vi "Main.vi"() -> ()   [LabVIEW 2018] (continued)
                n2123 = Delete From Array(array=w3655, length=w3654, index=62 ("索引")) -> (deleted portion=w3669:u32[])  [unwired: 1 out]
                n2124 = To Unsigned Word Integer(number=w3675) -> (unsigned 16bit integer=w3686:u16[])
                n2125 = To Unsigned Word Integer(number=w3676) -> (unsigned 16bit integer=w3677:u16[])
                n2126 = To Unsigned Word Integer(number=w3674) -> (unsigned 16bit integer=w3691:u16[])
                n2127 = To Unsigned Word Integer(number=w3656) -> (unsigned 16bit integer=w3661:u16[])
                n2128 = To Unsigned Word Integer(number=w3669) -> (unsigned 16bit integer=w3664:u16[])
                n2129 = call "还原为字符串.vi"("输入数组"=w3677) -> ("字符串"=w3679:string)  [unwired: 9 in, 1 out]
                n2130 = call "还原为字符串.vi"("输入数组"=w3686) -> ("字符串"=w3684:string)  [unwired: 9 in, 1 out]
                n2131 = call "还原为字符串.vi"("输入数组"=w3691) -> ("字符串"=w3689:string)  [unwired: 9 in, 1 out]
                n2132 = call "还原为字符串.vi"("输入数组"=w3661) -> ("字符串"=w3659:string)  [unwired: 9 in, 1 out]
                n2133 = call "还原为字符串.vi"("输入数组"=w3664) -> ("字符串"=w3666:string)  [unwired: 9 in, 1 out]
                n2134 = Match Pattern(string=w3679, regular expression="\r" ("正则表达式")) -> (before substring=w3678:string)  [unwired: 1 in, 3 out]
                n2135 = Match Pattern(string=w3684, regular expression="\r" ("正则表达式")) -> (before substring=w3685:string)  [unwired: 1 in, 3 out]
                n2136 = Match Pattern(string=w3689, regular expression="\r" ("正则表达式")) -> (before substring=w3690:string)  [unwired: 1 in, 3 out]
                n2137 = Match Pattern(string=w3659, regular expression="\r" ("正则表达式")) -> (before substring=w3660:string)  [unwired: 1 in, 3 out]
                n2138 = Match Pattern(string=w3666, regular expression="\r" ("正则表达式")) -> (before substring=w3665:string)  [unwired: 1 in, 3 out]
                n2139 = Match Pattern(string=w3678, regular expression="\u0000" ("正则表达式")) -> (before substring=w3653:string)  [unwired: 1 in, 3 out]
                n2140 = Match Pattern(string=w3685, regular expression="\u0000" ("正则表达式")) -> (before substring=w3652:string)  [unwired: 1 in, 3 out]
                n2141 = Match Pattern(string=w3690, regular expression="\u0000" ("正则表达式")) -> (before substring=w3651:string)  [unwired: 1 in, 3 out]
                n2142 = Match Pattern(string=w3660, regular expression="\u0000" ("正则表达式")) -> (before substring=w3649:string)  [unwired: 1 in, 3 out]
                n2143 = Match Pattern(string=w3665, regular expression="\u0000" ("正则表达式")) -> (before substring=w3650:string)  [unwired: 1 in, 3 out]
                n2144 = Insert Into Array(array=string[] [] ("数组"), index=0 ("索引"), new element #1="202" ("新元素/子数组"), new element #2=w3741, new element #3=w3739, new element #4=w3740, new element #5=w3741, new element #6=w3742, new element #7=w3743, new element #8=w3744, new element #9=w3745, new element #10=w3746, new element #11=w3747, new element #12=w3653, new element #13=w3652, new element #14=w3651, new element #15=w3650, new element #16=w3649) -> (w3647:string[])
                n2145 = stacked-sequence {
                  tunnel: w3670 -> [_ w3749]
                  tunnel: [_ w3750] -> w3648
                  tunnel: w3647 -> [w3748 _]
                  frame #0 {
                    "202data" <- w3748
                  }
                  frame #1 {
                    n2146 = property on="ST202数据读取(事件)" class="Bool (严格)"("Val(Sgnl)"=TRUE ("值(信号)")) -> ()  [unwired: 2 in, 2 out]
                    n2147 = disable-structure shown="禁用" {
                      disable-tunnel: w3749 -> [w3753 w3755]
                      disable-tunnel: [w3752 w3755] -> w3750
                      frame Disabled {
                        n2148 = property on="ST202画曲线" class="Bool (严格)"(error in=w3753, "Val(Sgnl)"=TRUE ("值(信号)")) -> (error out=w3752:errorcluster)  [unwired: 1 in, 1 out]
                      }
                      frame Enabled {
                      }
                    }
                  }
                }
              }
            }
          }
          frame "写" {
            w3914 = u8 132 items=["I/O (P)"=128, "Input (I)"=129, "Output (Q)"=130, "Bit Memory (M)"=131, "Data (DB)"=132, "Instance Data (DI)"=133, "Local Data (L)"=134, "Predecessor Local Data (VL)"=135] ("寄存器类型")
            w3913 = u16 1 items=["byte", "word", "Dword"] ("数据类型")
            w3931 = u8 132 items=["I/O (P)"=128, "Input (I)"=129, "Output (Q)"=130, "Bit Memory (M)"=131, "Data (DB)"=132, "Instance Data (DI)"=133, "Local Data (L)"=134, "Predecessor Local Data (VL)"=135] ("寄存器类型")
            w3932 = u16 1 items=["byte", "word", "Dword"] ("数据类型")
            w3939 = u8 132 items=["I/O (P)"=128, "Input (I)"=129, "Output (Q)"=130, "Bit Memory (M)"=131, "Data (DB)"=132, "Instance Data (DI)"=133, "Local Data (L)"=134, "Predecessor Local Data (VL)"=135] ("寄存器类型")
            w3940 = u16 1 items=["byte", "word", "Dword"] ("数据类型")
            w3942 = u8 132 items=["I/O (P)"=128, "Input (I)"=129, "Output (Q)"=130, "Bit Memory (M)"=131, "Data (DB)"=132, "Instance Data (DI)"=133, "Local Data (L)"=134, "Predecessor Local Data (VL)"=135] ("寄存器类型")
            w3941 = u16 1 items=["byte", "word", "Dword"] ("数据类型")
            w3948 = u8 132 items=["I/O (P)"=128, "Input (I)"=129, "Output (Q)"=130, "Bit Memory (M)"=131, "Data (DB)"=132, "Instance Data (DI)"=133, "Local Data (L)"=134, "Predecessor Local Data (VL)"=135] ("寄存器类型")
            w3945 = u16 1 items=["byte", "word", "Dword"] ("数据类型")
            n2149 = local read "20看门狗"() -> (w3924:i32)
            n2150 = case shown="0" w3924 {
              tunnel: [0 ("y") 1 ("y")] -> w3923
              frame 1, Default {
              }
              frame 0 {
              }
            }
            "20看门狗" <- w3923
            n2151 = call "S7_Write.vi"("TCP"=w3906, "寄存器类型"=w3948, "DB #"=u16 20, "写入地址"=u32 2, "数据类型"=w3945, "写入数据"=w3923) -> ("TCP"=w3922:refnum<k5>, "error out"=w3921:errorcluster)  [unwired: 7 in, 1 out]
            n2152 = case shown="假" "201扫码回复写入" {
              tunnel: w3922 -> [w3976 w3984]
              tunnel: w3921 -> [w3975 w3983]
              tunnel: [w3976 w3980] -> w3919
              tunnel: [w3975 w3979] -> w3918
              tunnel: [999 w3977] -> w3917
              frame False {
              }
              frame True {
                w3992 = u8 132 items=["I/O (P)"=128, "Input (I)"=129, "Output (Q)"=130, "Bit Memory (M)"=131, "Data (DB)"=132, "Instance Data (DI)"=133, "Local Data (L)"=134, "Predecessor Local Data (VL)"=135] ("寄存器类型")
                w3991 = u16 1 items=["byte", "word", "Dword"] ("数据类型")
                w3986 = u8 132 items=["I/O (P)"=128, "Input (I)"=129, "Output (Q)"=130, "Bit Memory (M)"=131, "Data (DB)"=132, "Instance Data (DI)"=133, "Local Data (L)"=134, "Predecessor Local Data (VL)"=135] ("寄存器类型")
                w3987 = u16 1 items=["byte", "word", "Dword"] ("数据类型")
                n2153 = local read "上一站号 (201)"() -> (w3982:string)
                n2154 = local read "上一站结果 (201)"() -> (w3981:string)
                n2155 = Decimal String To Number(string=w3982, default (0L)=u32 0 ("默认(0 I32)")) -> (number=w3996:u32)  [unwired: 1 in, 1 out]
                n2156 = call "S7_Write.vi"("TCP"=w3984, "寄存器类型"=w3986, "DB #"=u16 20, "写入地址"=u32 12, "数据类型"=w3987, "写入数据"=w3996, "error in"=w3983) -> ("TCP"=w3995:refnum<k5>, "error out"=w3994:errorcluster)  [unwired: 6 in, 1 out]
                n2157 = Equal?(x=w3981, y="OK") -> (x = y?=w3998:bool)
                n2158 = case shown="假" w3998 {
                  tunnel: [u32 2 ("写入数据") u32 1 ("写入数据")] -> w3999
                  frame False {
                  }
                  frame True {
                  }
                }
                n2159 = local read "扫码请求回复201"() -> (w3978:string)
                n2160 = call "S7_Write.vi"("TCP"=w3995, "寄存器类型"=w3992, "DB #"=u16 20, "写入地址"=u32 14, "数据类型"=w3991, "写入数据"=w3999, "error in"=w3994) -> ("TCP"=w3980:refnum<k5>, "error out"=w3979:errorcluster)  [unwired: 6 in, 1 out]
                n2161 = Decimal String To Number(string=w3978) -> (number=w3977:i32)  [unwired: 2 in, 1 out]
              }
            }
            n2162 = call "S7_Write.vi"("TCP"=w3919, "寄存器类型"=w3942, "DB #"=u16 20, "写入地址"=u32 4, "数据类型"=w3941, "写入数据"=w3917, "error in"=w3918) -> ("TCP"=w3912:refnum<k5>, "error out"=w3911:errorcluster)  [unwired: 6 in, 1 out]
            n2163 = case shown="真" "201数据回复写入" {
              tunnel: [999 w3972] -> w3910
              frame False {
              }
              frame True {
                n2164 = local read "数据保存请求回复201"() -> (w3973:string)
                n2165 = Decimal String To Number(string=w3973) -> (number=w3972:i32)  [unwired: 2 in, 1 out]
              }
            }
            n2166 = call "S7_Write.vi"("TCP"=w3912, "寄存器类型"=w3914, "DB #"=u16 20, "写入地址"=u32 6, "数据类型"=w3913, "写入数据"=w3910, "error in"=w3911) -> ("TCP"=w3908:refnum<k5>, "error out"=w3907:errorcluster)  [unwired: 6 in, 1 out]
            n2167 = case shown="真" "202扫码回复写入" {
              tunnel: [999 w4008] -> w3935
              tunnel: w3908 -> [w4006 w4025]
              tunnel: w3907 -> [w4005 w4024]
              tunnel: [w4006 w4013] -> w3934
              tunnel: [w4005 w4012] -> w3933
              frame False {
              }
              frame True {
                w4019 = u8 132 items=["I/O (P)"=128, "Input (I)"=129, "Output (Q)"=130, "Bit Memory (M)"=131, "Data (DB)"=132, "Instance Data (DI)"=133, "Local Data (L)"=134, "Predecessor Local Data (VL)"=135] ("寄存器类型")
                w4020 = u16 1 items=["byte", "word", "Dword"] ("数据类型")
                w4027 = u8 132 items=["I/O (P)"=128, "Input (I)"=129, "Output (Q)"=130, "Bit Memory (M)"=131, "Data (DB)"=132, "Instance Data (DI)"=133, "Local Data (L)"=134, "Predecessor Local Data (VL)"=135] ("寄存器类型")
                w4026 = u16 1 items=["byte", "word", "Dword"] ("数据类型")
                n2168 = local read "上一站号 (202)"() -> (w4011:string)
                n2169 = Decimal String To Number(string=w4011) -> (number=w4023:i32)  [unwired: 2 in, 1 out]
                n2170 = call "S7_Write.vi"("TCP"=w4025, "寄存器类型"=w4027, "DB #"=u16 20, "写入地址"=u32 16, "数据类型"=w4026, "写入数据"=w4023, "error in"=w4024) -> ("TCP"=w4015:refnum<k5>, "error out"=w4016:errorcluster)  [unwired: 6 in, 1 out]
                n2171 = local read "上一站结果 (202)"() -> (w4010:string)
                n2172 = local read "扫码请求回复202"() -> (w4009:string)
                n2173 = Equal?(x=w4010, y="OK") -> (x = y?=w4022:bool)
                n2174 = case shown="假" w4022 {
                  tunnel: [u32 2 ("写入数据") u32 1 ("写入数据")] -> w4014
                  frame False {
                  }
                  frame True {
                  }
                }
                n2175 = call "S7_Write.vi"("TCP"=w4015, "寄存器类型"=w4019, "DB #"=u16 20, "写入地址"=u32 18, "数据类型"=w4020, "写入数据"=w4014, "error in"=w4016) -> ("TCP"=w4013:refnum<k5>, "error out"=w4012:errorcluster)  [unwired: 6 in, 1 out]
                n2176 = Decimal String To Number(string=w4009) -> (number=w4008:i32)  [unwired: 2 in, 1 out]
              }
            }
            n2177 = call "S7_Write.vi"("TCP"=w3934, "寄存器类型"=w3939, "DB #"=u16 20, "写入地址"=u32 8, "数据类型"=w3940, "写入数据"=w3935, "error in"=w3933) -> ("TCP"=w3927:refnum<k5>, "error out"=w3928:errorcluster)  [unwired: 6 in, 1 out]
            n2178 = case shown="假" "202数据回复写入" {
              tunnel: [999 w4004] -> w3925
              frame False {
              }
              frame True {
                n2179 = local read "数据保存请求回复202"() -> (w4003:string)
                n2180 = Decimal String To Number(string=w4003) -> (number=w4004:i32)  [unwired: 2 in, 1 out]
              }
            }
            n2181 = call "S7_Write.vi"("TCP"=w3927, "寄存器类型"=w3931, "DB #"=u16 20, "写入地址"=u32 10, "数据类型"=w3932, "写入数据"=w3925, "error in"=w3928) -> ("TCP"=w3905:refnum<k5>, "error out"=w3903:errorcluster)  [unwired: 6 in, 1 out]
            n2182 = disable-structure shown="启用" {
              disable-tunnel: w3905 -> [w3951 w3967]
              disable-tunnel: [w3951 w3959] -> w3904
              disable-tunnel: w3903 -> [w3952 w3958]
              disable-tunnel: [w3952 w3956] -> w3902
              disable-tunnel: [_ w3954] -> w3901
              disable-tunnel: [_ w3953] -> w3900
              frame Disabled {
              }
              frame Enabled {
                w3965 = u16 20 ("DB #")
                w3964 = u8 132 items=["I/O (P)"=128, "Input (I)"=129, "Output (Q)"=130, "Bit Memory (M)"=131, "Data (DB)"=132, "Instance Data (DI)"=133, "Local Data (L)"=134, "Predecessor Local Data (VL)"=135] ("寄存器类型")
                w3963 = u16 1 items=["byte", "word", "Dword"] ("数据类型")
                n2183 = call "S7_Read.vi"("TCP"=w3967, "DB #"=w3965, "读取长度"=u16 1, "寄存器类型"=w3964, "起始地址"=u32 264 ("写入地址"), "数据类型"=w3963, "error in"=w3958) -> ("TCP"=w3966:refnum<k5>, "数据"=w3960:u32[], "error out"=w3957:errorcluster)  [unwired: 5 in, 1 out]
                n2184 = Index Array(array=w3960) -> (element=w3953:u32)  [unwired: 1 in]
                n2185 = case shown="1" w3953 {
                  tunnel: ["未选择" "LF37G" "LF37.1G"] -> w3954
                  frame 0, Default {
                  }
                  frame 1 {
                  }
                  frame 2 {
                  }
                }
                n2186 = call "S7_Write.vi"("TCP"=w3966, "寄存器类型"=w3964, "DB #"=w3965, "写入地址"=u32 266, "数据类型"=w3963, "写入数据"=w3953, "error in"=w3957) -> ("TCP"=w3959:refnum<k5>, "error out"=w3956:errorcluster)  [unwired: 6 in, 1 out]
              }
            }
            n2187 = local write "产品型号"(w3900) -> ()
            n2188 = local write "产品型号20-90"(w3901) -> ()
          }
          frame "错误" {
            n2189 = call "S7_Close.vi"("TCP Connection Ref"=w4036) -> ("error out"=w4037:errorcluster)  [unwired: 10 in]
            n2190 = call <vilib>:"Clear Errors.vi"("error in (no error)"=w4037) -> ()  [unwired: 5 in, 2 out]
          }
          frame "退出" {
            n2191 = call "S7_Close.vi"("TCP Connection Ref"=w4043) -> ("error out"=w4044:errorcluster)  [unwired: 10 in]
            n2192 = call <vilib>:"Clear Errors.vi"("error in (no error)"=w4044) -> ()  [unwired: 5 in, 2 out]
          }
        }
      }
      n2193 = while {
        shift-right: [w1194] -> _
        shift-left: errorcluster {"status"=FALSE, "code"=0, "source"=""} ("错误常量") -> [w1197]
        shift-right: [w1193] -> _
        shift-left: enum16{"初始化", "读", "写", "错误", "退出"}."初始化" -> [w1198]
        shift-right: [w1195] -> _
        shift-left: _ -> [w1192]
        stop <- w1191 stop-if-true
        n2194 = local read "退出"() -> (w1199:bool)
        n2195 = case shown="假" w1199 {
          tunnel: w1198 -> [w1200 _]
          tunnel: [w1201 enum16{"初始化", "读", "写", "错误", "退出"}."退出"] -> w1190
          tunnel: w1197 -> [w1202 _]
          frame False {
            n2196 = case shown="错误" w1202 {
              tunnel: [w1203 enum16{"初始化", "读", "写", "错误", "退出"}."错误"] -> w1201
              tunnel: w1200 -> [w1203 _]
              frame No Error {
              }
              frame Error {
              }
            }
          }
          frame True {
          }
        }
        n2197 = Wait (ms)(milliseconds to wait=u32 80 ("等待时间（毫秒）")) -> ()  [unwired: 1 out]
        n2198 = case shown="\"写\"" w1190 {
          tunnel: [w1206 w1258 w1567 refnum<k5> refnum ("TCP") refnum<k5> refnum ("TCP")] -> w1195
          tunnel: [w1207 w1257 w1565 errorcluster {"status"=FALSE, "code"=0, "source"=""} ("error out") errorcluster {"status"=FALSE, "code"=0, "source"=""} ("error out")] -> w1194
          tunnel: [enum16{"初始化", "读", "写", "错误", "退出"}."读" enum16{"初始化", "读", "写", "错误", "退出"}."写" enum16{"初始化", "读", "写", "错误", "退出"}."读" enum16{"初始化", "读", "写", "错误", "退出"}."初始化" enum16{"初始化", "读", "写", "错误", "退出"}."退出"] -> w1193
          tunnel: w1192 -> [_ w1289 w1625 w1738 w1745]
          tunnel: [FALSE FALSE FALSE FALSE TRUE] -> w1191
          frame "初始化", Default {
            w1219 = u16 0 items=["byte", "word", "Dword"] ("数据类型")
            w1217 = u8 132 items=["I/O (P)"=128, "Input (I)"=129, "Output (Q)"=130, "Bit Memory (M)"=131, "Data (DB)"=132, "Instance Data (DI)"=133, "Local Data (L)"=134, "Predecessor Local Data (VL)"=135] ("寄存器类型")
            w1230 = u16 0 items=["byte", "word", "Dword"] ("数据类型")
            w1232 = u8 132 items=["I/O (P)"=128, "Input (I)"=129, "Output (Q)"=130, "Bit Memory (M)"=131, "Data (DB)"=132, "Instance Data (DI)"=133, "Local Data (L)"=134, "Predecessor Local Data (VL)"=135] ("寄存器类型")
            w1221 = u16 0 items=["byte", "word", "Dword"] ("数据类型")
            w1223 = u8 132 items=["I/O (P)"=128, "Input (I)"=129, "Output (Q)"=130, "Bit Memory (M)"=131, "Data (DB)"=132, "Instance Data (DI)"=133, "Local Data (L)"=134, "Predecessor Local Data (VL)"=135] ("寄存器类型")
            w1245 = u8 0 items=["S7-1200.200.200SMART"=0, "S7-300"=2, "S7-400"=3] ("PLC 系列")
            n2199 = call "S7_Open.vi"("IP 地址"="192.168.1.60", "PLC 系列"=w1245, "超时（MS）"=100) -> ("TCP"=w1209:refnum<k5>, "error out"=w1208:errorcluster)  [unwired: 10 in, 1 out]
            n2200 = case shown="错误" w1208 {
              tunnel: [FALSE TRUE] -> w1241
              frame No Error {
              }
              frame Error {
              }
            }
            n2201 = local write "ST60通讯状态"(w1241) -> ()
            n2202 = call "S7_Read.vi"("TCP"=w1209, "DB #"=u16 20, "读取长度"=u16 13, "寄存器类型"=w1223, "起始地址"=u32 52, "数据类型"=w1221, "error in"=w1208) -> ("TCP"=w1238:refnum<k5>, "数据"=w1226:u32[], "error out"=w1228:errorcluster)  [unwired: 5 in, 1 out]
            n2203 = To Unsigned Word Integer(number=w1226) -> (unsigned 16bit integer=w1227:u16[])
            n2204 = call "还原为字符串.vi"("error in (no error)"=w1228, "输入数组"=w1227) -> ("error out"=w1239:errorcluster, "字符串"=w1229:string)  [unwired: 8 in]
            n2205 = local write "602二维码"(w1229) -> ()
            n2206 = call "S7_Read.vi"("TCP"=w1238, "DB #"=u16 20, "读取长度"=u16 13, "寄存器类型"=w1232, "起始地址"=u32 74, "数据类型"=w1230, "error in"=w1239) -> ("TCP"=w1211:refnum<k5>, "数据"=w1235:u32[], "error out"=w1237:errorcluster)  [unwired: 5 in, 1 out]
            n2207 = To Unsigned Word Integer(number=w1235) -> (unsigned 16bit integer=w1236:u16[])
            n2208 = call "还原为字符串.vi"("error in (no error)"=w1237, "输入数组"=w1236) -> ("error out"=w1210:errorcluster, "字符串"=w1240:string)  [unwired: 8 in]
            n2209 = local write "603二维码"(w1240) -> ()
            n2210 = call "S7_Read.vi"("TCP"=w1211, "DB #"=u16 20, "读取长度"=u16 13, "寄存器类型"=w1217, "起始地址"=u32 30, "数据类型"=w1219, "error in"=w1210) -> ("TCP"=w1206:refnum<k5>, "数据"=w1214:u32[], "error out"=w1212:errorcluster)  [unwired: 5 in, 1 out]
            n2211 = To Unsigned Word Integer(number=w1214) -> (unsigned 16bit integer=w1213:u16[])
            n2212 = call "还原为字符串.vi"("error in (no error)"=w1212, "输入数组"=w1213) -> ("error out"=w1207:errorcluster, "字符串"=w1220:string)  [unwired: 8 in]
            n2213 = local write "601二维码"(w1220) -> ()
          }
          frame "读" {
            w1290 = u16 0 items=["byte", "word", "Dword"] ("数据类型")
            w1292 = u8 132 items=["I/O (P)"=128, "Input (I)"=129, "Output (Q)"=130, "Bit Memory (M)"=131, "Data (DB)"=132, "Instance Data (DI)"=133, "Local Data (L)"=134, "Predecessor Local Data (VL)"=135] ("寄存器类型")
            n2214 = call "S7_Read.vi"("TCP"=w1289, "DB #"=u16 20, "读取长度"=u16 1, "寄存器类型"=w1292, "起始地址"=u32 0, "数据类型"=w1290) -> ("TCP"=w1287:refnum<k5>, "数据"=w1297:u32[], "读取成功"=w1300:bool, "error out"=w1286:errorcluster)  [unwired: 6 in]
            n2215 = Not(x=w1300) -> (.not. x?=→"ST60通讯状态":bool)
            n2216 = Index Array(array=w1297, index=0 ("索引")) -> (element=w1298:u32)
            n2217 = Number To Boolean Array(number=w1298) -> (Boolean array=w1299:bool[])
            n2218 = Index Array(array=w1299, index #1=0 ("索引")) -> (element #1=w1267:bool, element #2=w1256:bool, element #3=w1255:bool, element #4=w1252:bool, element #5=w1251:bool, element #6=w1249:bool)  [unwired: 5 in]
            "ST601扫码请求" <- w1267
            "ST601数据读取" <- w1256
            "ST602扫码请求" <- w1255
            "ST602数据读取" <- w1252
            "ST603扫码请求" <- w1251
            "ST603数据读取" <- w1249
            n2219 = disable-structure shown="启用" {
              disable-tunnel: [w1312 w1314] -> w1269
              disable-tunnel: w1267 -> [w1311 w1314]
              frame Disabled {
                n2220 = call <vilib>:"Boolean Crossing PtByPt.vi"("direction"=enum16{"either", "false-true", "true-false"}."true-false", "input"=w1311) -> ("crossing"=w1312:bool)  [unwired: 1 in]
              }
              frame Enabled {
              }
            }
            n2221 = call <vilib>:"Boolean Crossing PtByPt.vi"("direction"=enum16{"either", "false-true", "true-false"}."false-true", "input"=w1267) -> ("crossing"=w1285:bool)  [unwired: 1 in]
            n2222 = case shown="真" w1285 {
              tunnel: w1287 -> [w1546 w1551]
              tunnel: w1286 -> [w1545 w1552]
              tunnel: [w1546 w1550] -> w1284
              tunnel: [w1545 w1548] -> w1283
              frame False {
              }
              frame True {
                w1560 = u16 0 items=["byte", "word", "Dword"] ("数据类型")
                w1558 = u8 132 items=["I/O (P)"=128, "Input (I)"=129, "Output (Q)"=130, "Bit Memory (M)"=131, "Data (DB)"=132, "Instance Data (DI)"=133, "Local Data (L)"=134, "Predecessor Local Data (VL)"=135] ("寄存器类型")
                n2223 = call "S7_Read.vi"("TCP"=w1551, "DB #"=u16 20, "读取长度"=u16 13, "寄存器类型"=w1558, "起始地址"=u32 30, "数据类型"=w1560, "error in"=w1552) -> ("TCP"=w1550:refnum<k5>, "数据"=w1555:u32[], "error out"=w1553:errorcluster)  [unwired: 5 in, 1 out]
                n2224 = To Unsigned Word Integer(number=w1555) -> (unsigned 16bit integer=w1554:u16[])
                n2225 = call "还原为字符串.vi"("error in (no error)"=w1553, "输入数组"=w1554) -> ("error out"=w1549:errorcluster, "字符串"=w1547:string)  [unwired: 8 in]
                n2226 = stacked-sequence {
                  tunnel: w1549 -> [_ w1563]
                  tunnel: [_ w1562] -> w1548
                  tunnel: w1547 -> [w1561 _]
                  frame #0 {
                    "601二维码" <- w1561
                  }
                  frame #1 {
                    n2227 = property on="ST601扫码请求（事件）" class="Bool (严格)"(error in=w1563, "Val(Sgnl)"=TRUE ("值(信号)")) -> (error out=w1562:errorcluster)  [unwired: 1 in, 1 out]
                  }
                }
              }
            }
            n2228 = case shown="假" w1269 {
              frame False {
                n2229 = local write "601扫码回复输入"(FALSE ("301扫码回复输入")) -> ()
              }
              frame True {
              }
            }
            n2230 = call <vilib>:"Boolean Crossing PtByPt.vi"("direction"=enum16{"either", "false-true", "true-false"}."false-true", "input"=w1256) -> ("crossing"=w1281:bool)  [unwired: 1 in]
            n2231 = disable-structure shown="启用" {
              disable-tunnel: enum16{"either", "false-true", "true-false"}."true-false" ("direction") -> [w1325 _]
              disable-tunnel: [w1324 w1326] -> w1278
              disable-tunnel: w1256 -> [w1323 w1326]
              frame Disabled {
                n2232 = call <vilib>:"Boolean Crossing PtByPt.vi"("direction"=w1325, "input"=w1323) -> ("crossing"=w1324:bool)  [unwired: 1 in]
              }
              frame Enabled {
              }
            }
            n2233 = case shown="真" w1281 {
              tunnel: [w1505 w1515] -> w1276
              tunnel: [w1504 w1507] -> w1275
              tunnel: w1283 -> [w1504 w1511]
              tunnel: w1284 -> [w1505 w1512]
              frame False {
              }
              frame True {
                w1524 = u16 1 items=["byte", "word", "Dword"] ("数据类型")
                w1526 = u8 132 items=["I/O (P)"=128, "Input (I)"=129, "Output (Q)"=130, "Bit Memory (M)"=131, "Data (DB)"=132, "Instance Data (DI)"=133, "Local Data (L)"=134, "Predecessor Local Data (VL)"=135] ("寄存器类型")
                w1519 = u16 1 items=["byte", "word", "Dword"] ("数据类型")
                w1521 = u8 132 items=["I/O (P)"=128, "Input (I)"=129, "Output (Q)"=130, "Bit Memory (M)"=131, "Data (DB)"=132, "Instance Data (DI)"=133, "Local Data (L)"=134, "Predecessor Local Data (VL)"=135] ("寄存器类型")
                n2234 = call "S7_Read.vi"("TCP"=w1512, "DB #"=u16 20, "读取长度"=u16 1, "寄存器类型"=w1521, "起始地址"=u32 94, "数据类型"=w1519, "error in"=w1511) -> ("TCP"=w1532:refnum<k5>, "数据"=w1534:u32[], "error out"=w1533:errorcluster)  [unwired: 5 in, 1 out]
                n2235 = Index Array(array=w1534) -> (element=w1536:u32)  [unwired: 1 in]
                n2236 = Equal?(x=w1536, y=u32 1) -> (x = y?=w1535:bool)
                n2237 = case shown="真" w1535 {
                  tunnel: ["NG" "OK"] -> w1510
                  frame False {
                  }
                  frame True {
                  }
                }
                n2238 = call "S7_Read.vi"("TCP"=w1532, "DB #"=u16 20, "读取长度"=u16 1, "寄存器类型"=w1526, "起始地址"=u32 100, "数据类型"=w1524, "error in"=w1533) -> ("TCP"=w1515:refnum<k5>, "数据"=w1514:u32[], "error out"=w1508:errorcluster)  [unwired: 5 in, 1 out]
                n2239 = Index Array(array=w1514) -> (element=w1513:u32)  [unwired: 1 in]
                n2240 = Number To Decimal String(number=w1513) -> (decimal integer string=w1509:string)  [unwired: 1 in]
                n2241 = Format Date/Time String(time format string (%c)="%Y-%m-%d" ("时间格式字符串(%c)")) -> (date/time string=w1537:string)  [unwired: 2 in]
                n2242 = Get Date/Time String(want seconds? (F)=TRUE ("需要秒？(F)")) -> (time string=w1538:string)  [unwired: 2 in, 1 out]
                n2243 = Insert Into Array(array=string[] [] ("数组"), index=0 ("索引"), new element #1="601" ("新元素/子数组"), new element #2=w1510, new element #3=w1537, new element #4=w1538, new element #5=w1510, new element #6=w1509) -> (w1506:string[])
                n2244 = stacked-sequence {
                  tunnel: w1508 -> [_ w1542]
                  tunnel: [_ w1541] -> w1507
                  tunnel: w1506 -> [w1539 _]
                  frame #0 {
                    "601数据" <- w1539
                  }
                  frame #1 {
                    n2245 = property on="ST601数据读取（事件）" class="Bool (严格)"(error in=w1542, "Val(Sgnl)"=TRUE ("值(信号)")) -> (error out=w1541:errorcluster)  [unwired: 1 in, 1 out]
                  }
                }
              }
            }
            n2246 = case shown="假" w1278 {
              frame False {
                n2247 = local write "601数据回复输入"(FALSE ("301数据回复输入")) -> ()
              }
              frame True {
              }
            }
            n2248 = disable-structure shown="启用" {
              disable-tunnel: [w1309 w1310] -> w1277
              disable-tunnel: w1255 -> [w1307 w1310]
              frame Disabled {
                n2249 = call <vilib>:"Boolean Crossing PtByPt.vi"("direction"=enum16{"either", "false-true", "true-false"}."true-false", "input"=w1307) -> ("crossing"=w1309:bool)  [unwired: 1 in]
              }
              frame Enabled {
              }
            }
            n2250 = case shown="假" w1277 {
              frame False {
                n2251 = local write "602扫码回复输入"(FALSE ("302扫码回复输入")) -> ()
              }
              frame True {
              }
            }
            n2252 = disable-structure shown="启用" {
              disable-tunnel: [w1320 w1322] -> w1254
              disable-tunnel: w1252 -> [w1319 w1322]
              frame Disabled {
                n2253 = call <vilib>:"Boolean Crossing PtByPt.vi"("direction"=enum16{"either", "false-true", "true-false"}."true-false", "input"=w1319) -> ("crossing"=w1320:bool)  [unwired: 1 in]
              }
              frame Enabled {
              }
            }
            n2254 = case shown="假" w1254 {
              frame False {
                n2255 = local write "602数据回复输入"(FALSE ("302数据回复输入")) -> ()
              }
              frame True {
              }
            }
            n2256 = disable-structure shown="启用" {
              disable-tunnel: [w1305 w1306] -> w1253
              disable-tunnel: w1251 -> [w1303 w1306]
              frame Disabled {
                n2257 = call <vilib>:"Boolean Crossing PtByPt.vi"("direction"=enum16{"either", "false-true", "true-false"}."true-false", "input"=w1303) -> ("crossing"=w1305:bool)  [unwired: 1 in]
              }
              frame Enabled {
              }
            }
            n2258 = call <vilib>:"Boolean Crossing PtByPt.vi"("direction"=enum16{"either", "false-true", "true-false"}."false-true", "input"=w1255) -> ("crossing"=w1274:bool)  [unwired: 1 in]
            n2259 = case shown="真" w1274 {
              tunnel: w1276 -> [w1482 w1488]
              tunnel: w1275 -> [w1481 w1487]
              tunnel: [w1481 w1484] -> w1272
              tunnel: [w1482 w1486] -> w1273
              frame False {
              }
              frame True {
                w1489 = u16 0 items=["byte", "word", "Dword"] ("数据类型")
                w1491 = u8 132 items=["I/O (P)"=128, "Input (I)"=129, "Output (Q)"=130, "Bit Memory (M)"=131, "Data (DB)"=132, "Instance Data (DI)"=133, "Local Data (L)"=134, "Predecessor Local Data (VL)"=135] ("寄存器类型")
                n2260 = call "S7_Read.vi"("TCP"=w1488, "DB #"=u16 20, "读取长度"=u16 13, "寄存器类型"=w1491, "起始地址"=u32 52, "数据类型"=w1489, "error in"=w1487) -> ("TCP"=w1486:refnum<k5>, "数据"=w1494:u32[], "error out"=w1496:errorcluster)  [unwired: 5 in, 1 out]
                n2261 = To Unsigned Word Integer(number=w1494) -> (unsigned 16bit integer=w1495:u16[])
                n2262 = call "还原为字符串.vi"("error in (no error)"=w1496, "输入数组"=w1495) -> ("error out"=w1485:errorcluster, "字符串"=w1483:string)  [unwired: 8 in]
                n2263 = stacked-sequence {
                  tunnel: w1485 -> [_ w1500]
                  tunnel: [_ w1499] -> w1484
                  tunnel: w1483 -> [w1497 _]
                  frame #0 {
                    "602二维码" <- w1497
                  }
                  frame #1 {
                    n2264 = property on="ST602扫码请求 （事件）" class="Bool (严格)"(error in=w1500, "Val(Sgnl)"=TRUE ("值(信号)")) -> (error out=w1499:errorcluster)  [unwired: 1 in, 1 out]
                  }
                }
              }
            }
            n2265 = case shown="假" w1253 {
              frame False {
                n2266 = local write "603扫码回复输入"(FALSE ("303扫码回复输入")) -> ()
              }
              frame True {
              }
            }
            n2267 = disable-structure shown="启用" {
              disable-tunnel: [w1316 w1318] -> w1250
              disable-tunnel: w1249 -> [w1315 w1318]
              frame Disabled {
                n2268 = call <vilib>:"Boolean Crossing PtByPt.vi"("direction"=enum16{"either", "false-true", "true-false"}."true-false", "input"=w1315) -> ("crossing"=w1316:bool)  [unwired: 1 in]
              }
              frame Enabled {
              }
            }
            n2269 = case shown="假" w1250 {
              frame False {
                n2270 = local write "603数据回复输入"(FALSE ("303数据回复输入")) -> ()
              }
              frame True {
              }
            }
            n2271 = call <vilib>:"Boolean Crossing PtByPt.vi"("direction"=enum16{"either", "false-true", "true-false"}."false-true", "input"=w1252) -> ("crossing"=w1270:bool)  [unwired: 1 in]
            n2272 = case shown="真" w1270 {
              tunnel: w1273 -> [w1441 w1447]
              tunnel: w1272 -> [w1440 w1446]
              tunnel: [w1441 w1445] -> w1264
              tunnel: [w1440 w1443] -> w1263
              frame False {
              }
              frame True {
                w1453 = u16 1 items=["byte", "word", "Dword"] ("数据类型")
                w1455 = u8 132 items=["I/O (P)"=128, "Input (I)"=129, "Output (Q)"=130, "Bit Memory (M)"=131, "Data (DB)"=132, "Instance Data (DI)"=133, "Local Data (L)"=134, "Predecessor Local Data (VL)"=135] ("寄存器类型")
                w1448 = u16 1 items=["byte", "word", "Dword"] ("数据类型")
                w1450 = u8 132 items=["I/O (P)"=128, "Input (I)"=129, "Output (Q)"=130, "Bit Memory (M)"=131, "Data (DB)"=132, "Instance Data (DI)"=133, "Local Data (L)"=134, "Predecessor Local Data (VL)"=135] ("寄存器类型")
                n2273 = call "S7_Read.vi"("TCP"=w1447, "DB #"=u16 20, "读取长度"=u16 1, "寄存器类型"=w1450, "起始地址"=u32 102, "数据类型"=w1448, "error in"=w1446) -> ("TCP"=w1464:refnum<k5>, "数据"=w1466:u32[], "error out"=w1465:errorcluster)  [unwired: 5 in, 1 out]
                n2274 = Index Array(array=w1466) -> (element=w1467:u32)  [unwired: 1 in]
                n2275 = Number To Decimal String(number=w1467) -> (decimal integer string=w1474:string)  [unwired: 1 in]
                n2276 = call "S7_Read.vi"("TCP"=w1464, "DB #"=u16 20, "读取长度"=u16 1, "寄存器类型"=w1455, "起始地址"=u32 96, "数据类型"=w1453, "error in"=w1465) -> ("TCP"=w1445:refnum<k5>, "数据"=w1468:u32[], "error out"=w1444:errorcluster)  [unwired: 5 in, 1 out]
                n2277 = Index Array(array=w1468) -> (element=w1470:u32)  [unwired: 1 in]
                n2278 = Equal?(x=w1470, y=u32 1) -> (x = y?=w1469:bool)
                n2279 = case shown="真" w1469 {
                  tunnel: ["NG" "OK"] -> w1473
                  frame False {
                  }
                  frame True {
                  }
                }
                n2280 = Format Date/Time String(time format string (%c)="%Y-%m-%d" ("时间格式字符串(%c)")) -> (date/time string=w1471:string)  [unwired: 2 in]
                n2281 = Get Date/Time String(want seconds? (F)=TRUE ("需要秒？(F)")) -> (time string=w1472:string)  [unwired: 2 in, 1 out]
                n2282 = Insert Into Array(array=string[] [] ("数组"), index=0 ("索引"), new element #1="602" ("新元素/子数组"), new element #2=w1473, new element #3=w1471, new element #4=w1472, new element #5=w1473, new element #6=w1474) -> (w1442:string[])
                n2283 = stacked-sequence {
                  tunnel: w1444 -> [_ w1478]
                  tunnel: [_ w1477] -> w1443
                  tunnel: w1442 -> [w1475 _]
                  frame #0 {
                    "602data" <- w1475
                  }
                  frame #1 {
                    n2284 = property on="ST602数据读取（事件）" class="Bool (严格)"(error in=w1478, "Val(Sgnl)"=TRUE ("值(信号)")) -> (error out=w1477:errorcluster)  [unwired: 1 in, 1 out]
                  }
                }
              }
            }
            n2285 = call <vilib>:"Boolean Crossing PtByPt.vi"("direction"=enum16{"either", "false-true", "true-false"}."false-true", "input"=w1251) -> ("crossing"=w1266:bool)  [unwired: 1 in]
            n2286 = case shown="真" w1266 {
              tunnel: w1264 -> [w1421 w1427]
              tunnel: w1263 -> [w1420 w1426]
              tunnel: [w1420 w1423] -> w1259
              tunnel: [w1421 w1425] -> w1260
              frame False {
              }
              frame True {
                w1428 = u16 0 items=["byte", "word", "Dword"] ("数据类型")
                w1430 = u8 132 items=["I/O (P)"=128, "Input (I)"=129, "Output (Q)"=130, "Bit Memory (M)"=131, "Data (DB)"=132, "Instance Data (DI)"=133, "Local Data (L)"=134, "Predecessor Local Data (VL)"=135] ("寄存器类型")
                n2287 = call "S7_Read.vi"("TCP"=w1427, "DB #"=u16 20, "读取长度"=u16 13, "寄存器类型"=w1430, "起始地址"=u32 74, "数据类型"=w1428, "error in"=w1426) -> ("TCP"=w1425:refnum<k5>, "数据"=w1433:u32[], "error out"=w1435:errorcluster)  [unwired: 5 in, 1 out]
                n2288 = To Unsigned Word Integer(number=w1433) -> (unsigned 16bit integer=w1434:u16[])
                n2289 = call "还原为字符串.vi"("error in (no error)"=w1435, "输入数组"=w1434) -> ("error out"=w1424:errorcluster, "字符串"=w1422:string)  [unwired: 8 in]
                n2290 = stacked-sequence {
                  tunnel: w1424 -> [_ w1439]
                  tunnel: [_ w1438] -> w1423
                  tunnel: w1422 -> [w1436 _]
                  frame #0 {
                    "603二维码" <- w1436
                  }
                  frame #1 {
                    n2291 = property on="ST603扫码请求（事件）" class="Bool (严格)"(error in=w1439, "Val(Sgnl)"=TRUE ("值(信号)")) -> (error out=w1438:errorcluster)  [unwired: 1 in, 1 out]
                  }
                }
              }
            }
            n2292 = call <vilib>:"Boolean Crossing PtByPt.vi"("direction"=enum16{"either", "false-true", "true-false"}."false-true", "input"=w1249) -> ("crossing"=w1261:bool)  [unwired: 1 in]
            n2293 = case shown="真" w1261 {
              tunnel: w1260 -> [w1331 w1380]
              tunnel: w1259 -> [w1330 w1379]
              tunnel: [w1331 w1386] -> w1258
              tunnel: [w1330 w1333] -> w1257
              frame False {
              }
              frame True {
                w1348 = 15 ("长度")
                w1385 = u16 0 items=["byte", "word", "Dword"] ("数据类型")
                w1383 = u8 132 items=["I/O (P)"=128, "Input (I)"=129, "Output (Q)"=130, "Bit Memory (M)"=131, "Data (DB)"=132, "Instance Data (DI)"=133, "Local Data (L)"=134, "Predecessor Local Data (VL)"=135] ("寄存器类型")
                w1392 = u16 1 items=["byte", "word", "Dword"] ("数据类型")
                w1394 = u8 132 items=["I/O (P)"=128, "Input (I)"=129, "Output (Q)"=130, "Bit Memory (M)"=131, "Data (DB)"=132, "Instance Data (DI)"=133, "Local Data (L)"=134, "Predecessor Local Data (VL)"=135] ("寄存器类型")
                w1387 = u16 1 items=["byte", "word", "Dword"] ("数据类型")
                w1389 = u8 132 items=["I/O (P)"=128, "Input (I)"=129, "Output (Q)"=130, "Bit Memory (M)"=131, "Data (DB)"=132, "Instance Data (DI)"=133, "Local Data (L)"=134, "Predecessor Local Data (VL)"=135] ("寄存器类型")
                n2294 = call "S7_Read.vi"("TCP"=w1380, "DB #"=u16 20, "读取长度"=u16 100, "寄存器类型"=w1383, "起始地址"=u32 106, "数据类型"=w1385, "error in"=w1379) -> ("TCP"=w1378:refnum<k5>, "数据"=w1340:u32[], "error out"=w1377:errorcluster)  [unwired: 5 in, 1 out]
                n2295 = Delete From Array(array=w1340, length=w1348, index=2 ("索引")) -> (deleted portion=w1373:u32[])  [unwired: 1 out]
                n2296 = Delete From Array(array=w1340, length=w1348, index=22 ("索引")) -> (deleted portion=w1360:u32[])  [unwired: 1 out]
                n2297 = Delete From Array(array=w1340, length=w1348, index=42 ("索引")) -> (deleted portion=w1359:u32[])  [unwired: 1 out]
                n2298 = Delete From Array(array=w1340, length=w1348, index=62 ("索引")) -> (deleted portion=w1358:u32[])  [unwired: 1 out]
                n2299 = Delete From Array(array=w1340, length=w1348, index=82 ("索引")) -> (deleted portion=w1357:u32[])  [unwired: 1 out]
                n2300 = call "S7_Read.vi"("TCP"=w1378, "DB #"=u16 20, "读取长度"=u16 1, "寄存器类型"=w1389, "起始地址"=u32 104, "数据类型"=w1387, "error in"=w1377) -> ("TCP"=w1403:refnum<k5>, "数据"=w1405:u32[], "error out"=w1404:errorcluster)  [unwired: 5 in, 1 out]
                n2301 = To Unsigned Word Integer(number=w1360) -> (unsigned 16bit integer=w1370:u16[])
                n2302 = To Unsigned Word Integer(number=w1358) -> (unsigned 16bit integer=w1369:u16[])
                n2303 = To Unsigned Word Integer(number=w1373) -> (unsigned 16bit integer=w1376:u16[])
                n2304 = To Unsigned Word Integer(number=w1357) -> (unsigned 16bit integer=w1361:u16[])
                n2305 = To Unsigned Word Integer(number=w1359) -> (unsigned 16bit integer=w1364:u16[])
                n2306 = call "还原为字符串.vi"("输入数组"=w1376) -> ("字符串"=w1374:string)  [unwired: 9 in, 1 out]
                n2307 = call "还原为字符串.vi"("输入数组"=w1370) -> ("字符串"=w1372:string)  [unwired: 9 in, 1 out]
                n2308 = call "还原为字符串.vi"("输入数组"=w1364) -> ("字符串"=w1366:string)  [unwired: 9 in, 1 out]
                n2309 = call "还原为字符串.vi"("输入数组"=w1369) -> ("字符串"=w1367:string)  [unwired: 9 in, 1 out]
                n2310 = call "还原为字符串.vi"("输入数组"=w1361) -> ("字符串"=w1363:string)  [unwired: 9 in, 1 out]
                n2311 = Index Array(array=w1405) -> (element=w1406:u32)  [unwired: 1 in]
                n2312 = Number To Decimal String(number=w1406) -> (decimal integer string=w1413:string)  [unwired: 1 in]
                n2313 = Match Pattern(string=w1374, regular expression="\r" ("正则表达式")) -> (before substring=w1375:string)  [unwired: 1 in, 3 out]
                n2314 = Match Pattern(string=w1372, regular expression="\r" ("正则表达式")) -> (before substring=w1371:string)  [unwired: 1 in, 3 out]
                n2315 = Match Pattern(string=w1366, regular expression="\r" ("正则表达式")) -> (before substring=w1365:string)  [unwired: 1 in, 3 out]
                n2316 = Match Pattern(string=w1367, regular expression="\r" ("正则表达式")) -> (before substring=w1368:string)  [unwired: 1 in, 3 out]
                n2317 = Match Pattern(string=w1363, regular expression="\r" ("正则表达式")) -> (before substring=w1362:string)  [unwired: 1 in, 3 out]
                n2318 = call "S7_Read.vi"("TCP"=w1403, "DB #"=u16 20, "读取长度"=u16 1, "寄存器类型"=w1394, "起始地址"=u32 98, "数据类型"=w1392, "error in"=w1404) -> ("TCP"=w1386:refnum<k5>, "数据"=w1407:u32[], "error out"=w1334:errorcluster)  [unwired: 5 in, 1 out]
                n2319 = Index Array(array=w1407) -> (element=w1409:u32)  [unwired: 1 in]
                n2320 = Match Pattern(string=w1375, regular expression="\u0000" ("正则表达式")) -> (before substring=w1339:string)  [unwired: 1 in, 3 out]
                n2321 = Match Pattern(string=w1371, regular expression="\u0000" ("正则表达式")) -> (before substring=w1338:string)  [unwired: 1 in, 3 out]
                n2322 = Match Pattern(string=w1365, regular expression="\u0000" ("正则表达式")) -> (before substring=w1337:string)  [unwired: 1 in, 3 out]
                n2323 = Match Pattern(string=w1368, regular expression="\u0000" ("正则表达式")) -> (before substring=w1336:string)  [unwired: 1 in, 3 out]
                n2324 = Match Pattern(string=w1362, regular expression="\u0000" ("正则表达式")) -> (before substring=w1335:string)  [unwired: 1 in, 3 out]
                n2325 = Equal?(x=w1409, y=u32 1) -> (x = y?=w1408:bool)
                n2326 = case shown="真" w1408 {
                  tunnel: ["NG" "OK"] -> w1412
                  frame False {
                  }
                  frame True {
                  }
                }
                n2327 = Format Date/Time String(time format string (%c)="%Y-%m-%d" ("时间格式字符串(%c)")) -> (date/time string=w1410:string)  [unwired: 2 in]
                n2328 = Get Date/Time String(want seconds? (F)=TRUE ("需要秒？(F)")) -> (time string=w1411:string)  [unwired: 2 in, 1 out]
                n2329 = Insert Into Array(array=string[] [] ("数组"), index=0 ("索引"), new element #1="603" ("新元素/子数组"), new element #2=w1412, new element #3=w1410, new element #4=w1411, new element #5=w1412, new element #6=w1413, new element #7=w1339, new element #8=w1338, new element #9=w1337, new element #10=w1336, new element #11=w1335) -> (w1332:string[])
                n2330 = stacked-sequence {
                  tunnel: w1334 -> [_ w1417]
                  tunnel: [_ w1416] -> w1333
                  tunnel: w1332 -> [w1414 _]
                  frame #0 {
                    "603data" <- w1414
                  }
                  frame #1 {
                    n2331 = property on="ST603数据读取（事件）" class="Bool (严格)"(error in=w1417, "Val(Sgnl)"=TRUE ("值(信号)")) -> (error out=w1416:errorcluster)  [unwired: 1 in, 1 out]
                  }
                }
              }
            }
          }
          frame "写" {
            w1581 = u8 132 items=["I/O (P)"=128, "Input (I)"=129, "Output (Q)"=130, "Bit Memory (M)"=131, "Data (DB)"=132, "Instance Data (DI)"=133, "Local Data (L)"=134, "Predecessor Local Data (VL)"=135] ("寄存器类型")
            w1580 = u16 1 items=["byte", "word", "Dword"] ("数据类型")
            w1574 = u8 132 items=["I/O (P)"=128, "Input (I)"=129, "Output (Q)"=130, "Bit Memory (M)"=131, "Data (DB)"=132, "Instance Data (DI)"=133, "Local Data (L)"=134, "Predecessor Local Data (VL)"=135] ("寄存器类型")
            w1573 = u16 1 items=["byte", "word", "Dword"] ("数据类型")
            w1599 = u8 132 items=["I/O (P)"=128, "Input (I)"=129, "Output (Q)"=130, "Bit Memory (M)"=131, "Data (DB)"=132, "Instance Data (DI)"=133, "Local Data (L)"=134, "Predecessor Local Data (VL)"=135] ("寄存器类型")
            w1598 = u16 1 items=["byte", "word", "Dword"] ("数据类型")
            w1612 = u8 132 items=["I/O (P)"=128, "Input (I)"=129, "Output (Q)"=130, "Bit Memory (M)"=131, "Data (DB)"=132, "Instance Data (DI)"=133, "Local Data (L)"=134, "Predecessor Local Data (VL)"=135] ("寄存器类型")
            w1613 = u16 1 items=["byte", "word", "Dword"] ("数据类型")
            w1619 = u8 132 items=["I/O (P)"=128, "Input (I)"=129, "Output (Q)"=130, "Bit Memory (M)"=131, "Data (DB)"=132, "Instance Data (DI)"=133, "Local Data (L)"=134, "Predecessor Local Data (VL)"=135] ("寄存器类型")
            w1620 = u16 1 items=["byte", "word", "Dword"] ("数据类型")
            w1622 = u8 132 items=["I/O (P)"=128, "Input (I)"=129, "Output (Q)"=130, "Bit Memory (M)"=131, "Data (DB)"=132, "Instance Data (DI)"=133, "Local Data (L)"=134, "Predecessor Local Data (VL)"=135] ("寄存器类型")
            w1621 = u16 1 items=["byte", "word", "Dword"] ("数据类型")
            w1629 = u8 132 items=["I/O (P)"=128, "Input (I)"=129, "Output (Q)"=130, "Bit Memory (M)"=131, "Data (DB)"=132, "Instance Data (DI)"=133, "Local Data (L)"=134, "Predecessor Local Data (VL)"=135] ("寄存器类型")
            w1626 = u16 1 items=["byte", "word", "Dword"] ("数据类型")
            n2332 = local read "60看门狗"() -> (w1592:i32)
            n2333 = case shown="0" w1592 {
              tunnel: [0 ("y") 1 ("y")] -> w1591
              frame 1, Default {
              }
              frame 0 {
              }
            }
            "60看门狗" <- w1591
            n2334 = call "S7_Write.vi"("TCP"=w1625, "寄存器类型"=w1629, "DB #"=u16 20, "写入地址"=u32 2, "数据类型"=w1626, "写入数据"=w1591) -> ("TCP"=w1606:refnum<k5>, "error out"=w1605:errorcluster)  [unwired: 7 in, 1 out]
            n2335 = case shown="真" "601扫码回复输入" {
              tunnel: w1606 -> [w1678 w1686]
              tunnel: w1605 -> [w1677 w1685]
              tunnel: [w1678 w1684] -> w1604
              tunnel: [w1677 w1683] -> w1603
              tunnel: [999 w1682] -> w1602
              frame False {
              }
              frame True {
                w1694 = u8 132 items=["I/O (P)"=128, "Input (I)"=129, "Output (Q)"=130, "Bit Memory (M)"=131, "Data (DB)"=132, "Instance Data (DI)"=133, "Local Data (L)"=134, "Predecessor Local Data (VL)"=135] ("寄存器类型")
                w1693 = u16 1 items=["byte", "word", "Dword"] ("数据类型")
                w1688 = u8 132 items=["I/O (P)"=128, "Input (I)"=129, "Output (Q)"=130, "Bit Memory (M)"=131, "Data (DB)"=132, "Instance Data (DI)"=133, "Local Data (L)"=134, "Predecessor Local Data (VL)"=135] ("寄存器类型")
                w1689 = u16 1 items=["byte", "word", "Dword"] ("数据类型")
                n2336 = local read "上一站号 (601)"() -> (w1681:string)
                n2337 = local read "上一站结果 (601)"() -> (w1680:string)
                n2338 = Decimal String To Number(string=w1681, default (0L)=u32 0 ("默认(0 I32)")) -> (number=w1698:u32)  [unwired: 1 in, 1 out]
                n2339 = call "S7_Write.vi"("TCP"=w1686, "寄存器类型"=w1688, "DB #"=u16 20, "写入地址"=u32 16, "数据类型"=w1689, "写入数据"=w1698, "error in"=w1685) -> ("TCP"=w1697:refnum<k5>, "error out"=w1696:errorcluster)  [unwired: 6 in, 1 out]
                n2340 = Equal?(x=w1680, y="OK") -> (x = y?=w1700:bool)
                n2341 = case shown="假" w1700 {
                  tunnel: [u32 2 ("写入数据") u32 1 ("写入数据")] -> w1701
                  frame False {
                  }
                  frame True {
                  }
                }
                n2342 = local read "扫码请求回复601"() -> (w1679:string)
                n2343 = call "S7_Write.vi"("TCP"=w1697, "寄存器类型"=w1694, "DB #"=u16 20, "写入地址"=u32 18, "数据类型"=w1693, "写入数据"=w1701, "error in"=w1696) -> ("TCP"=w1684:refnum<k5>, "error out"=w1683:errorcluster)  [unwired: 6 in, 1 out]
                n2344 = Decimal String To Number(string=w1679) -> (number=w1682:i32)  [unwired: 2 in, 1 out]
              }
            }
            n2345 = call "S7_Write.vi"("TCP"=w1604, "寄存器类型"=w1622, "DB #"=u16 20, "写入地址"=u32 4, "数据类型"=w1621, "写入数据"=w1602, "error in"=w1603) -> ("TCP"=w1597:refnum<k5>, "error out"=w1596:errorcluster)  [unwired: 6 in, 1 out]
            n2346 = case shown="假" "601数据回复输入" {
              tunnel: [999 w1675] -> w1595
              frame False {
              }
              frame True {
                n2347 = local read "数据保存请求回复601"() -> (w1674:string)
                n2348 = Decimal String To Number(string=w1674) -> (number=w1675:i32)  [unwired: 2 in, 1 out]
              }
            }
            n2349 = call "S7_Write.vi"("TCP"=w1597, "寄存器类型"=w1599, "DB #"=u16 20, "写入地址"=u32 6, "数据类型"=w1598, "写入数据"=w1595, "error in"=w1596) -> ("TCP"=w1594:refnum<k5>, "error out"=w1593:errorcluster)  [unwired: 6 in, 1 out]
            n2350 = case shown="真" "602扫码回复输入" {
              tunnel: [999 w1713] -> w1616
              tunnel: w1594 -> [w1708 w1727]
              tunnel: w1593 -> [w1707 w1726]
              tunnel: [w1708 w1715] -> w1615
              tunnel: [w1707 w1714] -> w1614
              frame False {
              }
              frame True {
                w1721 = u8 132 items=["I/O (P)"=128, "Input (I)"=129, "Output (Q)"=130, "Bit Memory (M)"=131, "Data (DB)"=132, "Instance Data (DI)"=133, "Local Data (L)"=134, "Predecessor Local Data (VL)"=135] ("寄存器类型")
                w1722 = u16 1 items=["byte", "word", "Dword"] ("数据类型")
                w1729 = u8 132 items=["I/O (P)"=128, "Input (I)"=129, "Output (Q)"=130, "Bit Memory (M)"=131, "Data (DB)"=132, "Instance Data (DI)"=133, "Local Data (L)"=134, "Predecessor Local Data (VL)"=135] ("寄存器类型")
                w1728 = u16 1 items=["byte", "word", "Dword"] ("数据类型")
                n2351 = local read "上一站号 (602)"() -> (w1712:string)
                n2352 = Decimal String To Number(string=w1712) -> (number=w1725:i32)  [unwired: 2 in, 1 out]
                n2353 = call "S7_Write.vi"("TCP"=w1727, "寄存器类型"=w1729, "DB #"=u16 20, "写入地址"=u32 20, "数据类型"=w1728, "写入数据"=w1725, "error in"=w1726) -> ("TCP"=w1717:refnum<k5>, "error out"=w1718:errorcluster)  [unwired: 6 in, 1 out]
                n2354 = local read "上一站结果 (602)"() -> (w1711:string)
                n2355 = local read "扫码请求回复602"() -> (w1710:string)
                n2356 = Equal?(x=w1711, y="OK") -> (x = y?=w1724:bool)
                n2357 = case shown="假" w1724 {
                  tunnel: [u32 2 ("写入数据") u32 1 ("写入数据")] -> w1716
                  frame False {
                  }
                  frame True {
                  }
                }
                n2358 = call "S7_Write.vi"("TCP"=w1717, "寄存器类型"=w1721, "DB #"=u16 20, "写入地址"=u32 22, "数据类型"=w1722, "写入数据"=w1716, "error in"=w1718) -> ("TCP"=w1715:refnum<k5>, "error out"=w1714:errorcluster)  [unwired: 6 in, 1 out]
                n2359 = Decimal String To Number(string=w1710) -> (number=w1713:i32)  [unwired: 2 in, 1 out]
              }
            }
            n2360 = call "S7_Write.vi"("TCP"=w1615, "寄存器类型"=w1619, "DB #"=u16 20, "写入地址"=u32 8, "数据类型"=w1620, "写入数据"=w1616, "error in"=w1614) -> ("TCP"=w1608:refnum<k5>, "error out"=w1609:errorcluster)  [unwired: 6 in, 1 out]
            n2361 = case shown="假" "602数据回复输入" {
              tunnel: [999 w1706] -> w1607
              frame False {
              }
              frame True {
                n2362 = local read "数据保存请求回复602"() -> (w1705:string)
                n2363 = Decimal String To Number(string=w1705) -> (number=w1706:i32)  [unwired: 2 in, 1 out]
              }
            }
            n2364 = call "S7_Write.vi"("TCP"=w1608, "寄存器类型"=w1612, "DB #"=u16 20, "写入地址"=u32 10, "数据类型"=w1613, "写入数据"=w1607, "error in"=w1609) -> ("TCP"=w1572:refnum<k5>, "error out"=w1571:errorcluster)  [unwired: 6 in, 1 out]
            n2365 = case shown="真" "603扫码回复输入" {
              tunnel: [999 w1652] -> w1577
              tunnel: w1572 -> [w1647 w1666]
              tunnel: w1571 -> [w1646 w1665]
              tunnel: [w1647 w1654] -> w1578
              tunnel: [w1646 w1653] -> w1579
              frame False {
              }
              frame True {
                w1660 = u8 132 items=["I/O (P)"=128, "Input (I)"=129, "Output (Q)"=130, "Bit Memory (M)"=131, "Data (DB)"=132, "Instance Data (DI)"=133, "Local Data (L)"=134, "Predecessor Local Data (VL)"=135] ("寄存器类型")
                w1661 = u16 1 items=["byte", "word", "Dword"] ("数据类型")
                w1668 = u8 132 items=["I/O (P)"=128, "Input (I)"=129, "Output (Q)"=130, "Bit Memory (M)"=131, "Data (DB)"=132, "Instance Data (DI)"=133, "Local Data (L)"=134, "Predecessor Local Data (VL)"=135] ("寄存器类型")
                w1667 = u16 1 items=["byte", "word", "Dword"] ("数据类型")
                n2366 = local read "上一站号 (603)"() -> (w1650:string)
                n2367 = Decimal String To Number(string=w1650) -> (number=w1664:i32)  [unwired: 2 in, 1 out]
                n2368 = call "S7_Write.vi"("TCP"=w1666, "寄存器类型"=w1668, "DB #"=u16 20, "写入地址"=u32 24, "数据类型"=w1667, "写入数据"=w1664, "error in"=w1665) -> ("TCP"=w1656:refnum<k5>, "error out"=w1657:errorcluster)  [unwired: 6 in, 1 out]
                n2369 = local read "上一站结果 (603)"() -> (w1649:string)
                n2370 = Equal?(x=w1649, y="OK") -> (x = y?=w1663:bool)
                n2371 = local read "扫码请求回复603"() -> (w1651:string)
                n2372 = case shown="假" w1663 {
                  tunnel: [u32 2 ("写入数据") u32 1 ("写入数据")] -> w1655
                  frame False {
                  }
                  frame True {
                  }
                }
                n2373 = call "S7_Write.vi"("TCP"=w1656, "寄存器类型"=w1660, "DB #"=u16 20, "写入地址"=u32 26, "数据类型"=w1661, "写入数据"=w1655, "error in"=w1657) -> ("TCP"=w1654:refnum<k5>, "error out"=w1653:errorcluster)  [unwired: 6 in, 1 out]
                n2374 = Decimal String To Number(string=w1651) -> (number=w1652:i32)  [unwired: 2 in, 1 out]
              }
            }
            n2375 = call "S7_Write.vi"("TCP"=w1578, "寄存器类型"=w1574, "DB #"=u16 20, "写入地址"=u32 12, "数据类型"=w1573, "写入数据"=w1577, "error in"=w1579) -> ("TCP"=w1585:refnum<k5>, "error out"=w1584:errorcluster)  [unwired: 6 in, 1 out]
            n2376 = case shown="真" "603数据回复输入" {
              tunnel: [999 w1645] -> w1586
              frame False {
              }
              frame True {
                n2377 = local read "数据保存请求回复603"() -> (w1644:string)
                n2378 = Decimal String To Number(string=w1644) -> (number=w1645:i32)  [unwired: 2 in, 1 out]
              }
            }
            n2379 = call "S7_Write.vi"("TCP"=w1585, "寄存器类型"=w1581, "DB #"=u16 20, "写入地址"=u32 14, "数据类型"=w1580, "写入数据"=w1586, "error in"=w1584) -> ("TCP"=w1568:refnum<k5>, "error out"=w1566:errorcluster)  [unwired: 6 in, 1 out]
            n2380 = disable-structure shown="启用" {
              disable-tunnel: w1568 -> [w1632 w1636]
              disable-tunnel: [w1632 w1639] -> w1567
              disable-tunnel: w1566 -> [w1633 w1637]
              disable-tunnel: [w1633 w1638] -> w1565
              frame Disabled {
              }
              frame Enabled {
                w1641 = u8 132 items=["I/O (P)"=128, "Input (I)"=129, "Output (Q)"=130, "Bit Memory (M)"=131, "Data (DB)"=132, "Instance Data (DI)"=133, "Local Data (L)"=134, "Predecessor Local Data (VL)"=135] ("寄存器类型")
                w1635 = u16 1 items=["byte", "word", "Dword"] ("数据类型")
                n2381 = local read "产品型号"() -> (w1634:u32)
                n2382 = call "S7_Write.vi"("TCP"=w1636, "寄存器类型"=w1641, "DB #"=u16 20, "写入地址"=u32 206, "数据类型"=w1635, "写入数据"=w1634, "error in"=w1637) -> ("TCP"=w1639:refnum<k5>, "error out"=w1638:errorcluster)  [unwired: 6 in, 1 out]
              }
            }
          }
          frame "错误" {
            n2383 = call "S7_Close.vi"("TCP Connection Ref"=w1738) -> ("error out"=w1739:errorcluster)  [unwired: 10 in]
            n2384 = call <vilib>:"Clear Errors.vi"("error in (no error)"=w1739) -> ()  [unwired: 5 in, 2 out]
          }
          frame "退出" {
            n2385 = call "S7_Close.vi"("TCP Connection Ref"=w1745) -> ("error out"=w1746:errorcluster)  [unwired: 10 in]
            n2386 = call <vilib>:"Clear Errors.vi"("error in (no error)"=w1746) -> ()  [unwired: 5 in, 2 out]
          }
        }
      }
      n2387 = while {
        shift-right: [w213] -> _
        shift-left: errorcluster {"status"=FALSE, "code"=0, "source"=""} ("错误常量") -> [w216]
        shift-right: [w212] -> _
        shift-left: enum16{"初始化", "读", "写", "错误", "退出"}."初始化" -> [w217]
        shift-right: [w214] -> _
        shift-left: _ -> [w211]
        stop <- w210 stop-if-true
        n2388 = local read "退出"() -> (w218:bool)
        n2389 = case shown="假" w218 {
          tunnel: w217 -> [w219 _]
          tunnel: [w220 enum16{"初始化", "读", "写", "错误", "退出"}."退出"] -> w209
          tunnel: w216 -> [w221 _]
          frame False {
            n2390 = case shown="错误" w221 {
              tunnel: [w222 enum16{"初始化", "读", "写", "错误", "退出"}."错误"] -> w220
              tunnel: w219 -> [w222 _]
              frame No Error {
              }
              frame Error {
              }
            }
          }
          frame True {
          }
        }
        n2391 = Wait (ms)(milliseconds to wait=u32 80 ("等待时间（毫秒）")) -> ()  [unwired: 1 out]
        n2392 = case shown="\"写\"" w209 {
          tunnel: [w231 w289 w533 refnum<k5> refnum ("TCP") refnum<k5> refnum ("TCP")] -> w214
          tunnel: [w230 w288 w532 errorcluster {"status"=FALSE, "code"=0, "source"=""} ("error out") errorcluster {"status"=FALSE, "code"=0, "source"=""} ("error out")] -> w213
          tunnel: [enum16{"初始化", "读", "写", "错误", "退出"}."读" enum16{"初始化", "读", "写", "错误", "退出"}."写" enum16{"初始化", "读", "写", "错误", "退出"}."读" enum16{"初始化", "读", "写", "错误", "退出"}."初始化" enum16{"初始化", "读", "写", "错误", "退出"}."退出"] -> w212
          tunnel: w211 -> [_ w311 w584 w694 w701]
          tunnel: [FALSE FALSE FALSE FALSE TRUE] -> w210
          frame "初始化", Default {
            w242 = u16 0 items=["byte", "word", "Dword"] ("数据类型")
            w240 = u8 132 items=["I/O (P)"=128, "Input (I)"=129, "Output (Q)"=130, "Bit Memory (M)"=131, "Data (DB)"=132, "Instance Data (DI)"=133, "Local Data (L)"=134, "Predecessor Local Data (VL)"=135] ("寄存器类型")
            w252 = u16 0 items=["byte", "word", "Dword"] ("数据类型")
            w254 = u8 132 items=["I/O (P)"=128, "Input (I)"=129, "Output (Q)"=130, "Bit Memory (M)"=131, "Data (DB)"=132, "Instance Data (DI)"=133, "Local Data (L)"=134, "Predecessor Local Data (VL)"=135] ("寄存器类型")
            w244 = u16 0 items=["byte", "word", "Dword"] ("数据类型")
            w246 = u8 132 items=["I/O (P)"=128, "Input (I)"=129, "Output (Q)"=130, "Bit Memory (M)"=131, "Data (DB)"=132, "Instance Data (DI)"=133, "Local Data (L)"=134, "Predecessor Local Data (VL)"=135] ("寄存器类型")
            w267 = u8 0 items=["S7-1200.200.200SMART"=0, "S7-300"=2, "S7-400"=3] ("PLC 系列")
            n2393 = call "S7_Open.vi"("IP 地址"="192.168.1.90", "PLC 系列"=w267, "超时（MS）"=100) -> ("TCP"=w232:refnum<k5>, "error out"=w229:errorcluster)  [unwired: 10 in, 1 out]
            n2394 = case shown="错误" w229 {
              tunnel: [FALSE TRUE] -> w263
              frame No Error {
              }
              frame Error {
              }
            }
            n2395 = local write "ST90通讯状态"(w263) -> ()
            n2396 = call "S7_Read.vi"("TCP"=w232, "DB #"=u16 20, "读取长度"=u16 14, "寄存器类型"=w246, "起始地址"=u32 84, "数据类型"=w244, "error in"=w229) -> ("TCP"=w261:refnum<k5>, "数据"=w249:u32[], "error out"=w251:errorcluster)  [unwired: 5 in, 1 out]
            n2397 = To Unsigned Word Integer(number=w249) -> (unsigned 16bit integer=w250:u16[])
            n2398 = call "还原为字符串.vi"("error in (no error)"=w251, "输入数组"=w250) -> ("error out"=w262:errorcluster, "字符串"=w226:string)  [unwired: 8 in]
            n2399 = String To Byte Array(string=w226) -> (unsigned byte array=w227:u8[])
            n2400 = for {
              tunnel: w227 -> [w270] mode=indexing
              tunnel: [w269] -> w228 mode=indexing
              n2401 = Equal?(x=w270, y=u8 32) -> (x = y?=w271:bool)
              n2402 = case shown="真" w271 {
                tunnel: w270 -> [w273 _]
                tunnel: [w273 u8 48] -> w269
                frame False {
                }
                frame True {
                }
              }
            }
            n2403 = call "S7_Read.vi"("TCP"=w261, "DB #"=u16 20, "读取长度"=u16 13, "寄存器类型"=w254, "起始地址"=u32 146, "数据类型"=w252, "error in"=w262) -> ("TCP"=w234:refnum<k5>, "数据"=w257:u32[], "error out"=w259:errorcluster)  [unwired: 5 in, 1 out]
            n2404 = Byte Array To String(unsigned byte array=w228) -> (string=w225:string)
            n2405 = To Unsigned Word Integer(number=w257) -> (unsigned 16bit integer=w258:u16[])
            n2406 = local write "901编码"(w225) -> ()
            n2407 = call "还原为字符串.vi"("error in (no error)"=w259, "输入数组"=w258) -> ("error out"=w233:errorcluster, "字符串"=w260:string)  [unwired: 8 in]
            n2408 = local write "902二维码"(w260) -> ()
            n2409 = call "S7_Read.vi"("TCP"=w234, "DB #"=u16 20, "读取长度"=u16 13, "寄存器类型"=w240, "起始地址"=u32 6, "数据类型"=w242, "error in"=w233) -> ("TCP"=w231:refnum<k5>, "数据"=w237:u32[], "error out"=w235:errorcluster)  [unwired: 5 in, 1 out]
            n2410 = To Unsigned Word Integer(number=w237) -> (unsigned 16bit integer=w236:u16[])
            n2411 = call "还原为字符串.vi"("error in (no error)"=w235, "输入数组"=w236) -> ("error out"=w230:errorcluster, "字符串"=w243:string)  [unwired: 8 in]
            n2412 = local write "901二维码"(w243) -> ()
          }
          frame "读" {
            w312 = u16 0 items=["byte", "word", "Dword"] ("数据类型")
            w314 = u8 132 items=["I/O (P)"=128, "Input (I)"=129, "Output (Q)"=130, "Bit Memory (M)"=131, "Data (DB)"=132, "Instance Data (DI)"=133, "Local Data (L)"=134, "Predecessor Local Data (VL)"=135] ("寄存器类型")
            n2413 = call "S7_Read.vi"("TCP"=w311, "DB #"=u16 20, "读取长度"=u16 1, "寄存器类型"=w314, "起始地址"=u32 0, "数据类型"=w312) -> ("TCP"=w309:refnum<k5>, "数据"=w319:u32[], "读取成功"=w322:bool, "error out"=w308:errorcluster)  [unwired: 6 in]
